vi "Detect Text (Greyscale).vi"(8 "error in (no error)":errorcluster, 10 "Greyscale Image in":T4, 11 "Text Detector in":refnum<class "Text Detector.lvclass">) -> (0 "error out":errorcluster, 2 "Detections":T1[](array[typedef]), 3 "Text Detector":refnum<class "Text Detector.lvclass">)   [LabVIEW 2020, in "feature_detection.lvlib" / "Text Detector.lvclass"]
uses:
  Text Detector.lvclass
  Text Detector.lvclass/Text Detector.ctl
  47bc948f-a394-4876-8faa-d1ac59be58fd.vi
  common/Image Point (Float).ctl
  common/common.lvlib
  common/Quad Corners.ctl
  Detection.ctl
  image/Greyscale Image.ctl
  image/image.lvlib
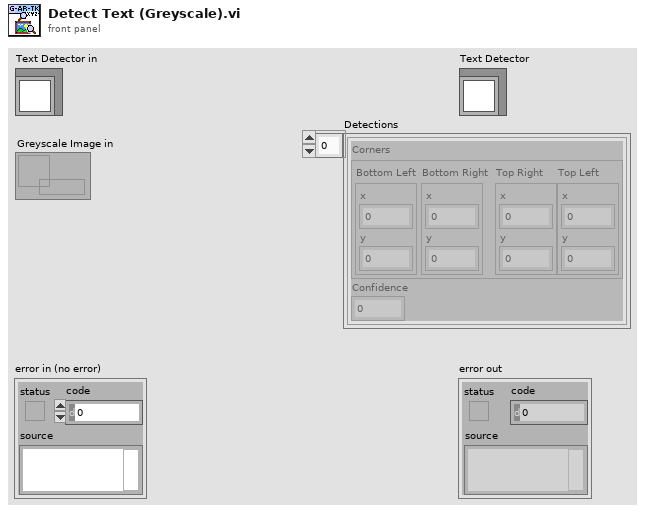
[diagram p1: front panel]
types:
  T1 = typedef "feature_detection.lvlib/Text Detector.lvclass/Detection.ctl" = cluster{"Corners":T2, "Confidence":sgl}
  T2 = typedef "common.lvlib/Quad Corners.ctl" = cluster{"Bottom Left":T3, "Bottom Right":T3, "Top Right":T3, "Top Left":T3}
  T3 = typedef "common.lvlib/Image Point (Float).ctl" = cluster{"x":dbl, "y":dbl}
  T4 = typedef "image.lvlib/Greyscale Image.ctl" = refnum<data-value>
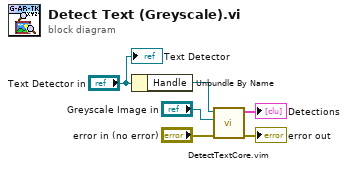
[diagram p0: block diagram]
diagram:
  n1 = Unbundle By Name("Text Detector in") -> ("Handle"=w4:refnum<data-value>)
  n2 = call "DetectTextCore.vim"("error in (no error)"="error in (no error)", "Greyscale Image in"="Greyscale Image in", "Detector in"=w4) -> ("error out"=→"error out":errorcluster, "Detections"=→"Detections":T1[])  [unwired: 7 in]
  "Text Detector" <- "Text Detector in"
